vi "FAseLockin.vi"(3 "error in (no error)":errorcluster) -> (0 "error out":errorcluster, 1 "Fase AFM":dbl, 2 "Fase NSOM":dbl)   [LabVIEW 2018]
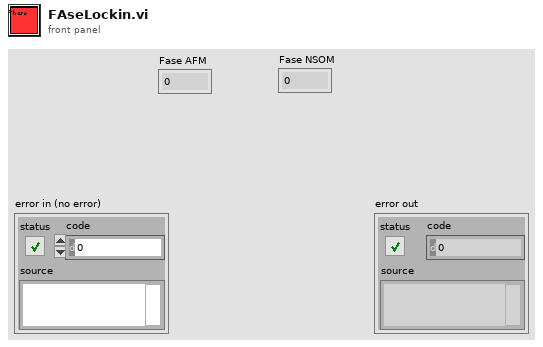
[diagram p1: front panel]
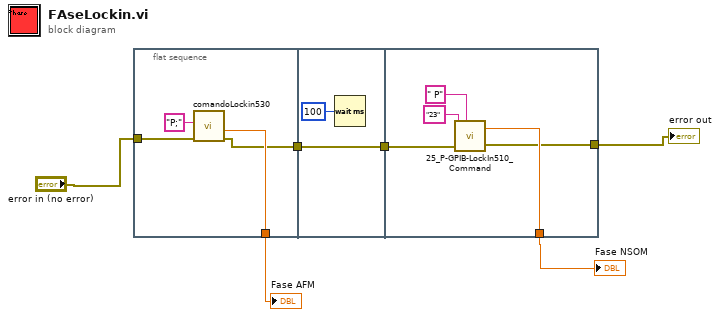
[diagram p0: block diagram]
diagram:
  n1 = flat-sequence {
    tunnel: [w9] -> w2
    tunnel: [w8] -> w6
    tunnel: "error in (no error)" -> [w7]
    tunnel: w6 -> [w11]
    tunnel: [w11] -> w5
    tunnel: w5 -> [w17]
    tunnel: [w14] -> w1
    tunnel: [w13] -> w3
    frame #0 {
      n2 = call "comandoLockin530.vi"("error in"=w7, "Comando"="P;") -> ("error out"=w8:errorcluster, "Fase"=w9:dbl)  [unwired: 8 in]
    }
    frame #1 {
      n3 = Wait (ms)(milliseconds to wait=u32 100) -> ()  [unwired: 1 out]
    }
    frame #2 {
      n4 = call "25_P-GPIB-LockIn510_Command.vi"("P-LockIn"="23", "Command"=" P", "error in (no error)"=w17) -> ("LockIn"=w14:dbl, "error out"=w13:errorcluster)  [unwired: 2 in]
    }
  }
  "Fase AFM" <- w2
  "Fase NSOM" <- w1
  "error out" <- w3
